vi "Data Logger Class Chooser.vi"(8 "error in (no error)":errorcluster, 11 "Generic Instrument.lvlib:Generic Instrument.lvclass":refnum<class "Generic Instrument.lvclass">) -> (0 "error out":errorcluster, 3 "Generic Instrument out":refnum<class "Generic Instrument.lvclass">)   [LabVIEW 2013, in "Generic Data Logger.lvlib" / "Generic Data Logger.lvclass"]
uses:
  Generic Data Logger.lvclass
  Generic Instrument/Generic Instrument.lvclass
  Generic Instrument/Generic Instrument.lvclass/Generic Instrument.ctl
panel:
  out "Boolean":bool
  out "Number of Cards":dbl
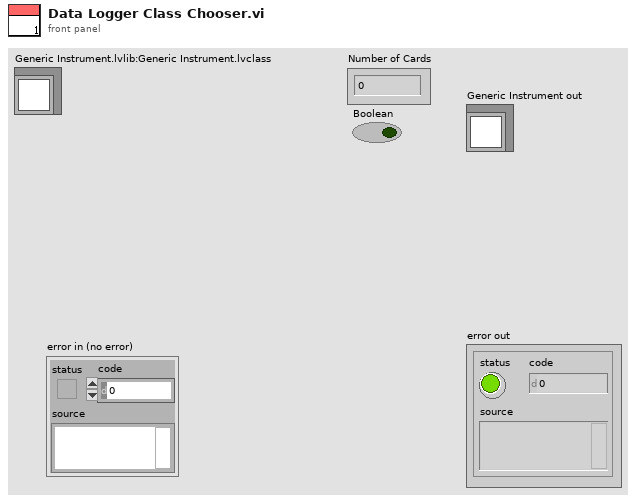
[diagram p1: front panel]
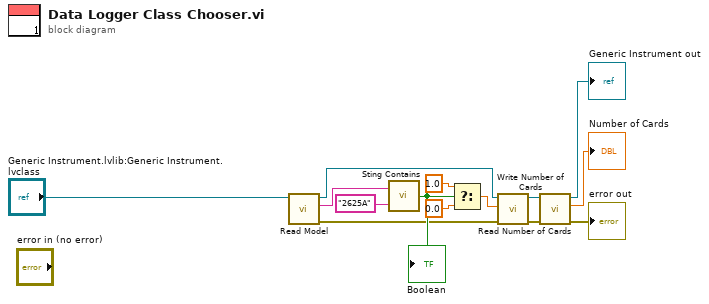
[diagram p0: block diagram]
diagram:
  n1 = call "Read Model.vi"("Generic Instrument in"="Generic Instrument.lvlib:Generic Instrument.lvclass") -> ("error out"=w6:errorcluster, "Model"=w13:string, "Generic Instrument out"=w7:refnum<class "Generic Instrument.lvclass">)  [unwired: 8 in]
  n2 = call "Sting Contains.vi"("Expression to evaluate"="2625A", "Input String"=w13) -> ("Boolean"=w11:bool)
  "Boolean" <- w11
  n3 = Select(t=1.0, s=w11, f=0.0) -> (s? t:f=w8:dbl)
  n4 = call-dynamic "Write Number of Cards.vi"("error in (no error)"=w6, "Number of Cards"=w8, "Generic Instrument in"=w7) -> ("error out"=w3:errorcluster, "Generic Instrument out"=w5:refnum<class "Generic Instrument.lvclass">)  [unwired: 7 in]
  n5 = call-dynamic "Read Number of Cards.vi"("error in (no error)"=w3, "Generic Instrument in"=w5) -> ("error out"=→"error out":errorcluster, "Number of Cards"=→"Number of Cards":dbl, "Generic Instrument out"=→"Generic Instrument out":refnum<class "Generic Instrument.lvclass">)  [unwired: 7 in]
